vi "SendPacket.vi"(8 "error in":errorcluster, 10 "Ethernet Port Opened ?":bool, 11 "Packet Array":string[](array[string])) -> (0 "error out":errorcluster, 3 "Time per plane":u32)   [LabVIEW 2017]
panel:
  out "Ethernet Port Open":bool
  out "FOR Loop":i32
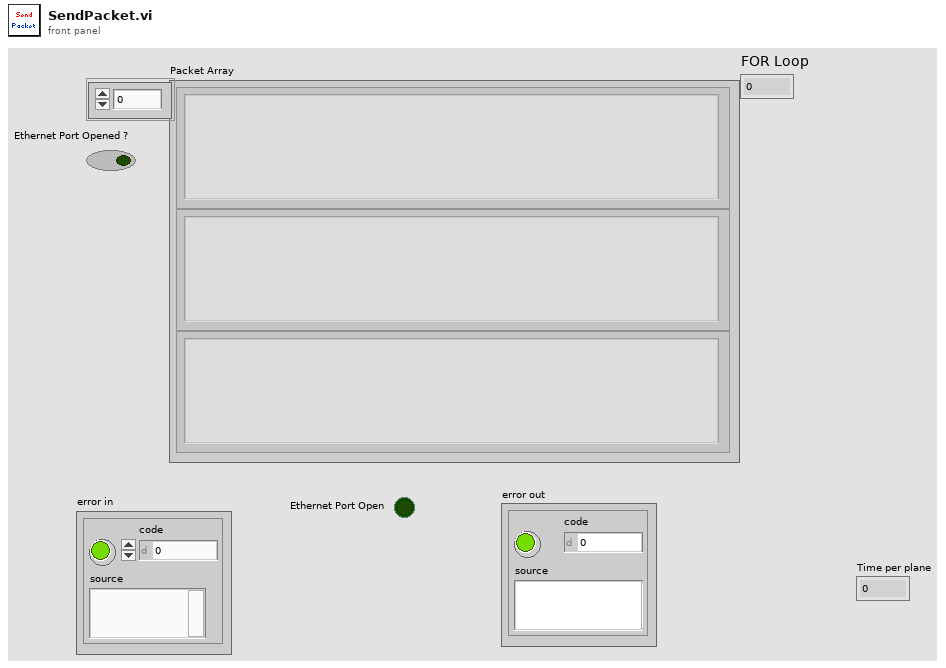
[diagram p1: front panel]
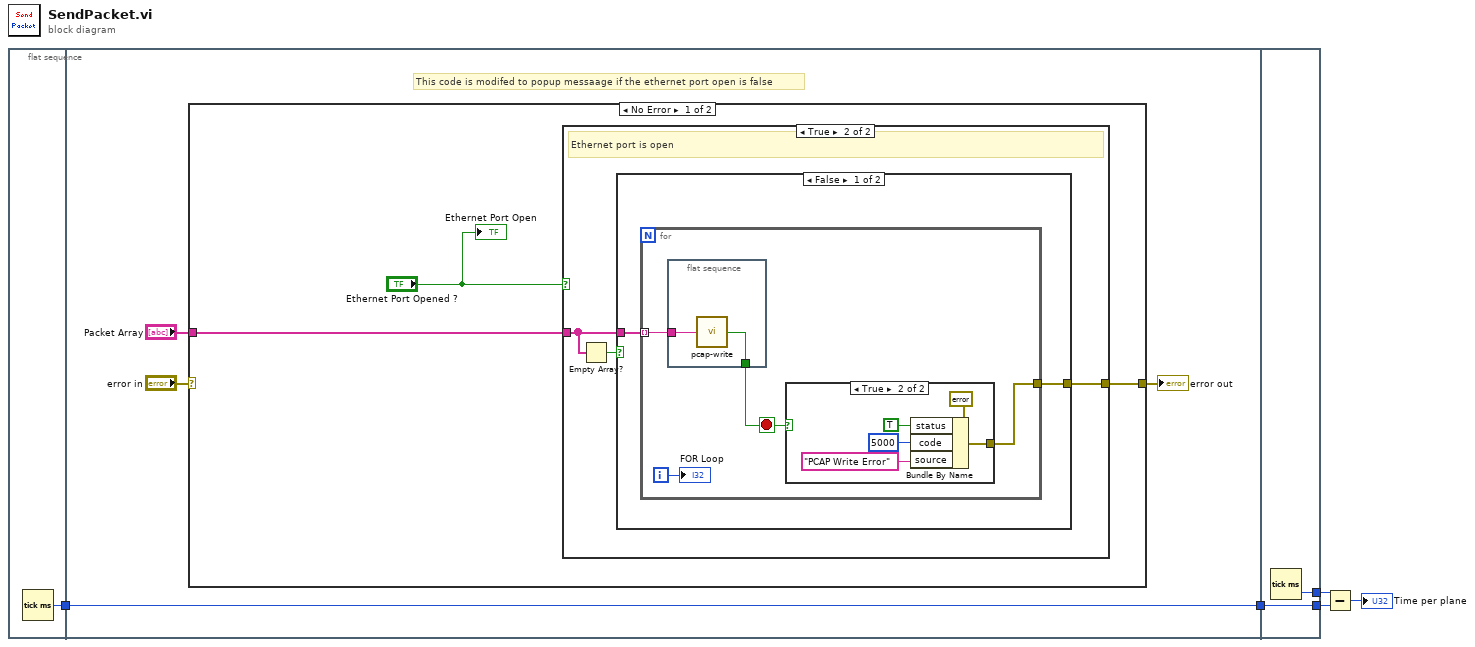
[diagram p0: block diagram]
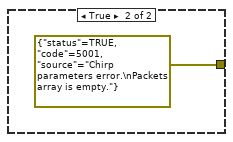
[diagram p4: hidden frame]
diagram:
  n1 = flat-sequence {
    tunnel: [w6] -> w4
    tunnel: w4 -> [w7]
    tunnel: [w7] -> w3
    tunnel: [w33] -> w5
    tunnel: w3 -> [w32]
    tunnel: [w32] -> w2
    frame #0 {
      n2 = Tick Count (ms)() -> (millisecond timer value=w6:u32)
    }
    frame #1 {
      # "This code is modifed to popup messaage if the ethernet port open is false"
      n3 = case shown="No Error" "error in" {
        selector: "error in" -> [_ w31]
        tunnel: "Packet Array" -> [w12 _]
        tunnel: [w13 w31] -> w9
        frame No Error {
          n4 = case shown="True" "Ethernet Port Opened ?" {
            tunnel: [_ w16] -> w13
            tunnel: w12 -> [_ w15]
            frame False {
              # "Ethernet port is closed"
            }
            frame True {
              # "Ethernet port is open"
              n5 = Empty Array?(array=w15) -> (empty?=w14:bool)
              n6 = case shown="False" w14 {
                tunnel: w15 -> [w18 _]
                tunnel: [w17 errorcluster {"status"=TRUE, "code"=5001, "source"="Chirp parameters error.\nPackets array is empty."} ("error out")] -> w16
                frame False {
                  n7 = for {
                    tunnel: w18 -> [w22] mode=indexing
                    tunnel: [w20] -> w17
                    i -> [w21]
                    stop <- w19 stop-if-true
                    n8 = flat-sequence {
                      tunnel: [w29] -> w19
                      tunnel: w22 -> [w28]
                      frame #0 {
                        n9 = call "pcap-write.vi"("Data to Write"=w28) -> ("Write Error"=w29:bool)
                      }
                    }
                    n10 = case shown="True" w19 {
                      tunnel: [_ w25] -> w20
                      frame False {
                      }
                      frame True {
                        n11 = Bundle By Name(cluster=errorcluster {"status"=FALSE, "code"=0, "source"=""} ("error out"), "status"=TRUE, "code"=5000, "source"="PCAP Write Error") -> (w25:errorcluster)
                      }
                    }
                    "FOR Loop" <- w21
                  }
                }
                frame True {
                }
              }
            }
          }
          "Ethernet Port Open" <- "Ethernet Port Opened ?"
        }
        frame Error {
        }
      }
      "error out" <- w9
    }
    frame #2 {
      n12 = Tick Count (ms)() -> (millisecond timer value=w33:u32)
    }
  }
  n13 = Subtract(x=w5, y=w2) -> (x-y=→"Time per plane":u32)
